vi "janelaTempoVI.vi"() -> ()   [LabVIEW 2014]
uses:
  <vilib>/MakerHub/LINX/Public/Peripherals/Digital/Digital Write 1 Chan.vi
  <vilib>/MakerHub/LINX/Public/Peripherals/Digital/Digital Write N Chans.vi
  <vilib>/MakerHub/LINX/Private/Local IO/LinxDigitalWrite.vi
  <vilib>/MakerHub/LINX/Public/Utilities/Check Channel.vi
  <vilib>/MakerHub/LINX/Private/Local IO/Handle Errors.vi
  <vilib>/MakerHub/LINX/Public/Utilities/Open Local.vi
  <vilib>/MakerHub/LINX/Private/Utilties/Generate Error.vi
  <vilib>/MakerHub/LINX/LMH-LINX.lvlib
panel:
  out "indicador de inicio":bool
  out "Interações":i32
  in  "Porta de inicio":u8
  out "Erro":T1
  in  "Porta da janela":u8
  in  "Iniciar Estudo":bool
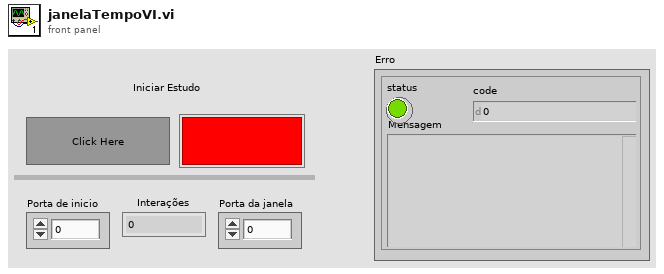
[diagram p1: front panel]
types:
  T1 = cluster{"status":bool, "code":i32, "Mensagem":string}
  T2 = typedef "LMH-LINX.lvlib/LINX Ref.ctl" = cluster{"IO":T3, "Interface":T4, "LINX Device Config":T5}
  T3 = typedef "LMH-LINX.lvlib/Platform.ctl" = enum16{"Remote", "Local"}
  T4 = typedef "LMH-LINX.lvlib/Interface.ctl" = enum16{"Serial", "TCP"}
  T5 = typedef "LMH-LINX.lvlib/Device.lvlib/LINX Device Config.ctl" = cluster{"Interface":T4, "COM Port":refnum<visa-resource-name>, "TCP Configuration":T6, "Device Family":u8, "Device ID":u8, "Device Name":string, "TCP Ref":refnum<k5>, "Channels":T7}
  T6 = typedef "LMH-LINX.lvlib/Device.lvlib/TCP Config.ctl" = cluster{"IP Address":string, "Port":u16}
  T7 = typedef "LMH-LINX.lvlib/Channels.ctl" = cluster{"DI":u8[], "DO":u8[], "AI":u8[], "AO":u8[], "PWM":u8[], "QE":u8[], "UART":u8[], "I2C 2":u8[], "SPI":u8[], "CAN":u8[], "Servo":u8[], "AI Ref (V)":dbl, "AI Resolution (Bits)":u8, "AO Ref (V)":dbl, "AO Resolution (Bits)":u8}
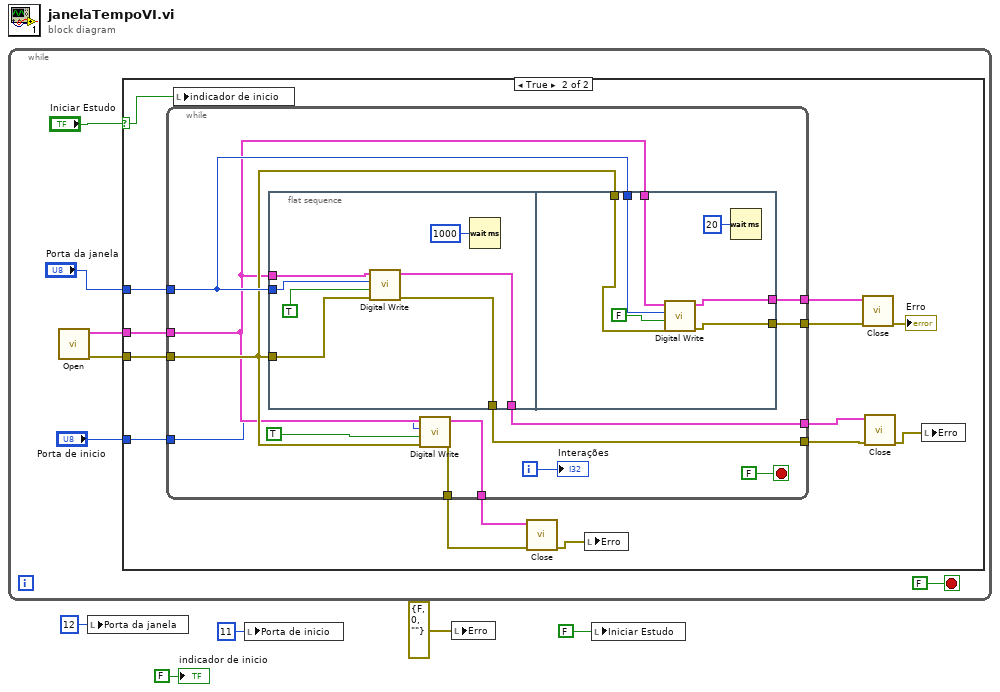
[diagram p0: block diagram]
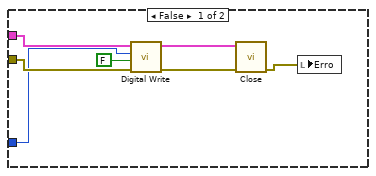
[diagram p2: hidden frame]
diagram:
  n1 = while {
    stop <- FALSE stop-if-true
    n2 = call-poly <vilib>:"Open.vi"() -> ("Error Out"=w7:errorcluster, "LINX Resource"=w9:T2)  [unwired: 9 in, 1 out]
    n3 = case shown="True" "Iniciar Estudo" {
      selector: "Iniciar Estudo" -> [_ w19]
      tunnel: w9 -> [w18 w32]
      tunnel: "Porta da janela" -> [_ w31]
      tunnel: w7 -> [w17 w30]
      tunnel: "Porta de inicio" -> [w13 w20]
      frame False {
        n4 = call-poly <vilib>:"Digital Write.vi"("Error In"=w17, "Output Value"=FALSE, "DO Channel"=w13, "LINX Resource"=w18) -> ("Error Out"=w15:errorcluster, "LINX Resource"=w16:T2)  [unwired: 6 in]
        n5 = call <vilib>:"Close.vi"("Error In"=w15, "LINX Resource"=w16) -> ("Error Out"=w14:errorcluster)  [unwired: 9 in]
        n6 = local write "Erro"(w14) -> ()
      }
      frame True {
        n7 = while {
          tunnel: w32 -> [w41]
          tunnel: w31 -> [w45]
          tunnel: w30 -> [w42]
          tunnel: [w44] -> w29
          tunnel: [w43] -> w28
          tunnel: [w39] -> w26
          tunnel: [w38] -> w25
          tunnel: [w37] -> w23
          tunnel: [w36] -> w22
          tunnel: w20 -> [w35]
          i -> [w34]
          stop <- FALSE stop-if-true
          n8 = flat-sequence {
            tunnel: w41 -> [w52]
            tunnel: w45 -> [w51]
            tunnel: w42 -> [w50]
            tunnel: [w47] -> w39
            tunnel: [w46] -> w38
            tunnel: w41 -> [w57]
            tunnel: w45 -> [w56]
            tunnel: w42 -> [w55]
            tunnel: [w54] -> w44
            tunnel: [w53] -> w43
            frame #0 {
              n9 = call-poly <vilib>:"Digital Write.vi"("Error In"=w50, "Output Value"=TRUE, "DO Channel"=w51, "LINX Resource"=w52) -> ("Error Out"=w46:errorcluster, "LINX Resource"=w47:T2)  [unwired: 6 in]
              n10 = Wait (ms)(milliseconds to wait=u32 1000) -> ()  [unwired: 1 out]
            }
            frame #1 {
              n11 = call-poly <vilib>:"Digital Write.vi"("Error In"=w55, "Output Value"=FALSE, "DO Channel"=w56, "LINX Resource"=w57) -> ("Error Out"=w53:errorcluster, "LINX Resource"=w54:T2)  [unwired: 6 in]
              n12 = Wait (ms)(milliseconds to wait=u32 20) -> ()  [unwired: 1 out]
            }
          }
          n13 = call-poly <vilib>:"Digital Write.vi"("Error In"=w42, "Output Value"=TRUE, "DO Channel"=w35, "LINX Resource"=w41) -> ("Error Out"=w36:errorcluster, "LINX Resource"=w37:T2)  [unwired: 6 in]
          "Interações" <- w34
        }
        n14 = local write "indicador de inicio"(w19) -> ()
        n15 = call <vilib>:"Close.vi"("Error In"=w22, "LINX Resource"=w23) -> ("Error Out"=w21:errorcluster)  [unwired: 9 in]
        n16 = local write "Erro"(w21) -> ()
        n17 = call <vilib>:"Close.vi"("Error In"=w28, "LINX Resource"=w29) -> ("Error Out"=→"Erro":errorcluster)  [unwired: 9 in]
        n18 = call <vilib>:"Close.vi"("Error In"=w25, "LINX Resource"=w26) -> ("Error Out"=w24:errorcluster)  [unwired: 9 in]
        n19 = local write "Erro"(w24) -> ()
      }
    }
  }
  n20 = local write "Porta da janela"(u8 12 ("Porta da janela")) -> ()
  n21 = local write "Porta de inicio"(u8 11 ("Porta de inicio")) -> ()
  n22 = local write "Erro"(errorcluster {"status"=FALSE, "code"=0, "source"=""} ("Error Out")) -> ()
  n23 = local write "Iniciar Estudo"(FALSE ("Janela de Tempo")) -> ()
  "indicador de inicio" <- FALSE ("indicador de inicio")
